vi "20220107_03.vi"   [LabVIEW 2019]
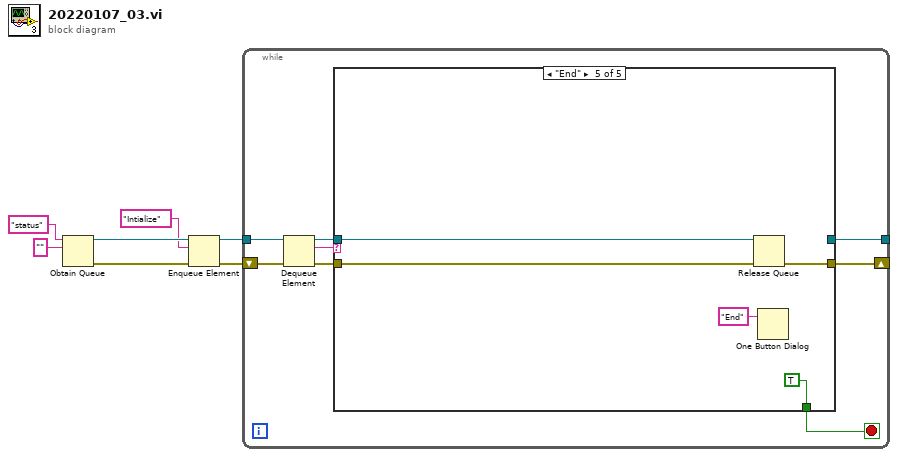
[diagram p0: block diagram]
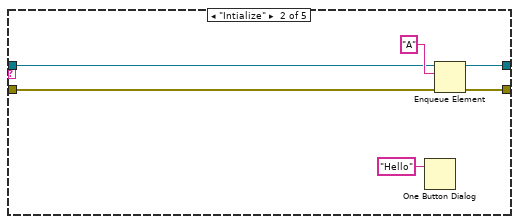
[diagram p3: hidden frame]
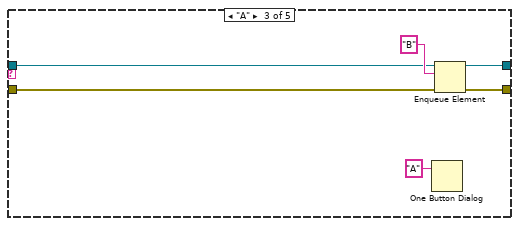
[diagram p4: hidden frame]
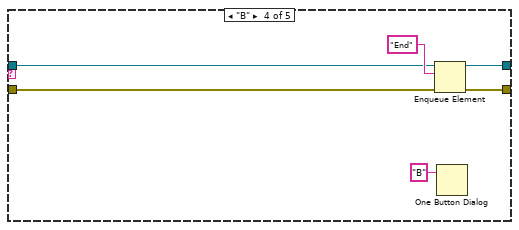
[diagram p5: hidden frame]
diagram:
  n1 = Obtain Queue(name (unnamed)="status", element data type="" ("name (unnamed)")) -> (queue out=w6:refnum<queue>, error out=w7:errorcluster)  [unwired: 3 in, 1 out]
  n2 = Enqueue Element(queue=w6, element="Intialize", error in (no error)=w7) -> (queue out=w1:refnum<queue>, error out=w2:errorcluster)  [unwired: 1 in, 1 out]
  n3 = while {
    shift-right: [w11] -> _
    shift-left: w2 -> [w15]
    tunnel: w1 -> [w14]
    tunnel: [w9] -> _
    stop <- w8 stop-if-true
    n4 = Dequeue Element(queue=w14, error in (no error)=w15) -> (queue out=w10:refnum<queue>, element=w12:string, error out=w13:errorcluster)  [unwired: 1 in, 1 out]
    n5 = case shown="\"End\"" w12 {
      tunnel: w13 -> [w17 w22 w28 w34 w40]
      tunnel: [w17 w19 w25 w31 w39] -> w11
      tunnel: w10 -> [w16 w21 w27 w33 w38]
      tunnel: [w16 w20 w26 w32 _] -> w9
      tunnel: [_ _ _ _ TRUE] -> w8
      frame Default {
      }
      frame "Intialize" {
        n6 = One Button Dialog(message="Hello") -> ()  [unwired: 1 in, 1 out]
        n7 = Enqueue Element(queue=w21, element="A", error in (no error)=w22) -> (queue out=w20:refnum<queue>, error out=w19:errorcluster)  [unwired: 1 in, 1 out]
      }
      frame "A" {
        n8 = One Button Dialog(message="A") -> ()  [unwired: 1 in, 1 out]
        n9 = Enqueue Element(queue=w27, element="B", error in (no error)=w28) -> (queue out=w26:refnum<queue>, error out=w25:errorcluster)  [unwired: 1 in, 1 out]
      }
      frame "B" {
        n10 = Enqueue Element(queue=w33, element="End", error in (no error)=w34) -> (queue out=w32:refnum<queue>, error out=w31:errorcluster)  [unwired: 1 in, 1 out]
        n11 = One Button Dialog(message="B") -> ()  [unwired: 1 in, 1 out]
      }
      frame "End" {
        n12 = Release Queue(queue=w38, error in (no error)=w40) -> (error out=w39:errorcluster)  [unwired: 1 in, 2 out]
        n13 = One Button Dialog(message="End") -> ()  [unwired: 1 in, 1 out]
      }
    }
  }
